vi "фронтовой RSDC-триггер.vi"(2 "S":bool, 3 "C":bool, 4 "D":bool, 5 "R":bool) -> (0 "not Q":bool, 1 "Q":bool)   [LabVIEW 2012]
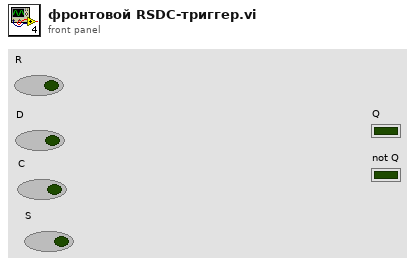
[diagram p1: front panel]
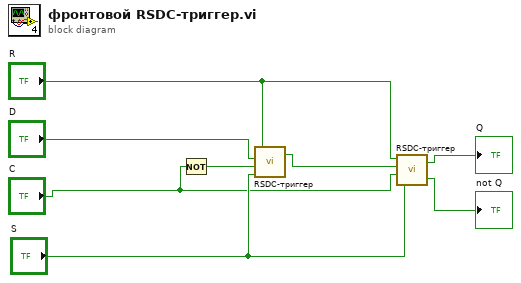
[diagram p0: block diagram]
diagram:
  n1 = Not(x="C") -> (.not. x?=w2:bool)
  n2 = call "RSDC-триггер.vi"("S"="S", "C"=w2, "D"="D", "R"="R") -> ("Q"=w8:bool)  [unwired: 1 out]
  n3 = call "RSDC-триггер.vi"("S"="S", "C"="C", "D"=w8, "R"="R") -> ("not Q"=→"not Q":bool, "Q"=→"Q":bool)
